vi "Init.vi"(8 "error in (no error)":errorcluster, 10 "Instrument String":variant, 11 "NI Fgen in":refnum<class "NI Fgen.lvclass">) -> (0 "error out":errorcluster, 2 "Found?":bool, 3 "NI Fgen out":refnum<class "NI Fgen.lvclass">)   [LabVIEW 2025, in "Fgen.lvlib" / "NI Fgen.lvclass"]
uses:
  NI Fgen.lvclass
  <instrlib>/niFgen/niFgen.llb/niFgen Output Mode.ctl
  Fgen configuration/Fgen configuration.lvclass
  Fgen configuration/Fgen configuration.lvclass/Fgen configuration.ctl
  NI Fgen.lvclass/NI Fgen.ctl
  Fgen configuration/Read Fgen Setting.vi
  Users/Public/Documents/Sandia National Labs/TSS Plugin/Abstract Engine.lvlibp/Plugin/Abstract/Instrument configuration/Read Instrument Setting.vi
  Users/Public/Documents/Sandia National Labs/TSS Plugin/CEF.lvlibp/serializable configuration/CEF_serializable configuration.lvclass
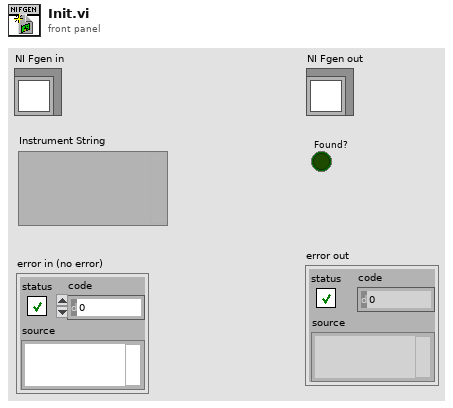
[diagram p1: front panel]
types:
  T1 = typedef "niFgen Output Mode.ctl" = u32
  T2 = typedef "Fgen.lvlib/Fgen configuration.lvclass/Fgen Setting.ctl" = cluster{"Type":string, "Output Mode":string, "Sample Rate":dbl, "Samples":dbl, "Gain":dbl, "Trigger":string, "Impedance":string, "Offset":dbl}
  T3 = cluster{"Type":string, "Engine IP Address":string, "Engine Port":u32, "Address":string, "SW Alias":string, "Description":string, "Enabled":bool, "Model":string, "Serial Number":string, "Asset Number":string, "Calibration Date":string}
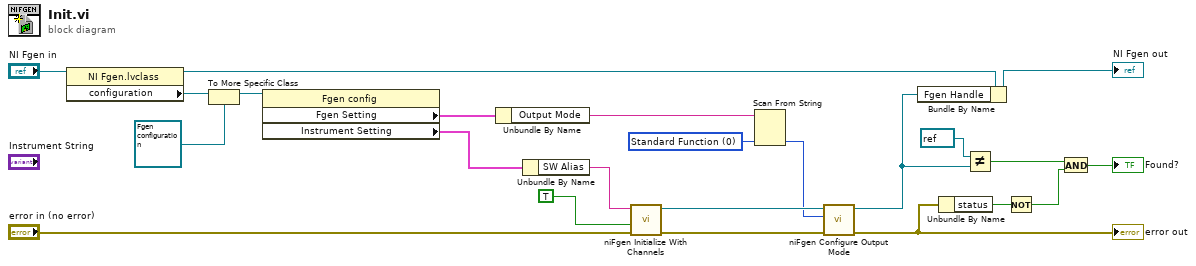
[diagram p0: block diagram]
diagram:
  w12 = T1 0 items=["Standard Function", "Frequency List", "Arbitrary Waveform", "Arbitrary Sequence", "Script"] ("Output Mode (default: 0=Standard Function)")
  n1 = property class="NI Fgen.lvclass"(reference="NI Fgen in") -> (reference out=w5:refnum<class "NI Fgen.lvclass">, "configuration"=w17:refnum<class "CEF_serializable configuration.lvclass">)  [unwired: 1 in, 1 out]
  n2 = To More Specific Class(target class=refnum<class "Fgen configuration.lvclass"> refnum ("Fgen.lvlib:Fgen configuration.lvclass"), reference=w17) -> (specific class reference=w16:refnum<class "Fgen configuration.lvclass">)  [unwired: 1 in, 1 out]
  n3 = property class="Fgen config"(reference=w16) -> ("Fgen Setting"=w2:T2, "Instrument Setting"=w3:T3)  [unwired: 1 in, 2 out]
  n4 = Unbundle By Name(w2) -> ("Output Mode"=w1:string)
  n5 = Unbundle By Name(w3) -> ("SW Alias"=w18:string)
  n6 = call <instrlib>:"niFgen Initialize With Channels.vi"("error in (no error)"="error in (no error)", "Reset Device (default: True)"=TRUE ("ID Query (True)"), "Resource Name"=w18) -> ("error out"=w15:errorcluster, "Instrument Handle Out"=w14:refnum<k15>)  [unwired: 7 in]
  n7 = Scan From String(input string=w1, default 1=w12) -> (output 1=w11:T1)  [unwired: 3 in, 3 out]
  n8 = call <instrlib>:"niFgen Configure Output Mode.vi"("error in (no error)"=w15, "Output Mode (default: 0=Standard Function)"=w11, "Instrument Handle"=w14) -> ("error out"=w9:errorcluster, "Instrument Handle Out"=w13:refnum<k15>)  [unwired: 6 in]
  "error out" <- w9
  n9 = Bundle By Name(cluster=w5, "Fgen Handle"=w13) -> (→"NI Fgen out":refnum<class "NI Fgen.lvclass">)
  n10 = Unbundle By Name(w9) -> ("status"=w10:bool)
  n11 = Not Equal?(x=refnum<k15> refnum ("Instrument Handle Out"), y=w13) -> (x != y?=w8:bool)
  n12 = Not(x=w10) -> (.not. x?=w7:bool)
  n13 = And(x=w8, y=w7) -> (x .and. y?=→"Found?":bool)
